vi "Report Pong.vi"(8 "error in (no error)":errorcluster, 11 "Keepalive Heartbeat in":refnum<class "Keepalive Heartbeat.lvclass">) -> (0 "error out":errorcluster, 3 "Keepalive Heartbeat out":refnum<class "Keepalive Heartbeat.lvclass">)   [LabVIEW 2021, in "WebSocket Actors.lvlib" / "Keepalive Heartbeat.lvclass"]
uses:
  Keepalive Heartbeat.lvclass
  Keepalive Heartbeat.lvclass/Keepalive Heartbeat.ctl
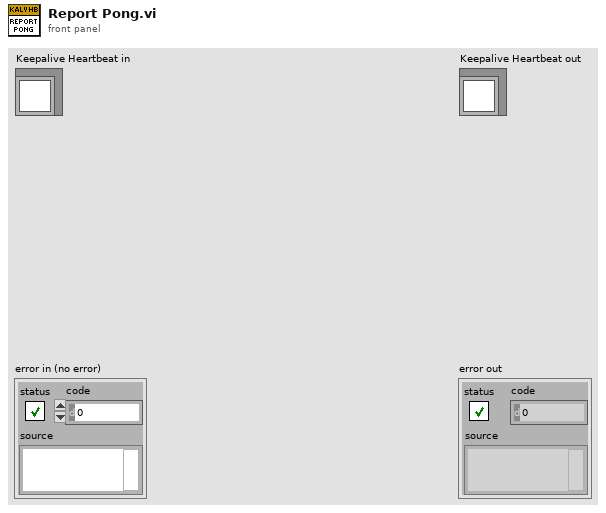
[diagram p1: front panel]
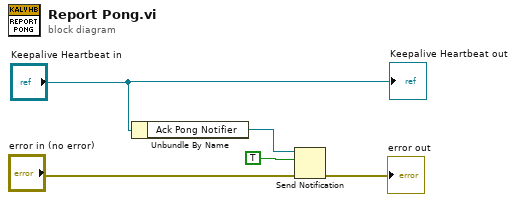
[diagram p0: block diagram]
diagram:
  n1 = Unbundle By Name("Keepalive Heartbeat in") -> ("Ack Pong Notifier"=w4:refnum<notifier>)
  n2 = Send Notification(notification=TRUE, notifier=w4, error in (no error)="error in (no error)") -> (error out=→"error out":errorcluster)  [unwired: 1 out]
  "Keepalive Heartbeat out" <- "Keepalive Heartbeat in"
